vi "PSK_Error_Analysis.vi"() -> ()   [LabVIEW 2014]
uses:
  <vilib>/addons/Modulation/Digital/General/MT Generate Bits (Galois, PN Order).vi
  <vilib>/addons/Modulation/Digital/Support/Common/Validators/mod_Generate Bits Validate.vi
  <vilib>/addons/Modulation/Analog/support/mod_Set Error Source.vi
  <vilib>/addons/Modulation/Digital/General/subVIs/mod_Generate Bits PN Sequence.vi
  <vilib>/addons/Modulation/niDMT.lvlib
panel:
  in  "Packet Parameters in":T1={"Length of sync sequence (50)"=50, "Number of message bits"=128, "Number of guardbits"=40, "Sync PN sequence order (31)"=31, "Number of header bits"=16, "Packet Pad [samples]"=0}
  out "Sync Errors":i32
  out "Bit Error Rate":dbl
  out "Payload bits transfered":i32
  in  "Test Setup":T2={"Iterations"=100, "Tx IQ Sampling\nRate [s/sec]"=400000.0} {"Tx IQ Sampling\nRate [s/sec]" format="%#.6p"}
  in  "Impairments":T3={"Delay (samples)"=9, "Eb/N0 (10 dB)"=10.0} {"Eb/N0 (10 dB)" format="%.2f"}
  out "Bit errors":i64
  out "Waveform Graph":cluster{"t0":dbl, "dt":dbl, "Y":dbl[]}[](graph)
  out "Packet Length (bits)":i32
  out "Max Xcorr Index Delayed":i32
  in  "PN sequence order (9)":i32=9 caption="Message PN sequence order"
  out "Frame Offset (measured)":i32
  out "output bit stream 2":i8[](array[numeric]) caption="Transmitted Packet"
  out "output bit stream":i8[](array[numeric]) caption="Received Packet"
  in  "filter parameters":T4={"Alpha"=0.5, "Filter Length"=6, "TX Filter"=enum."Root Raised Cos"} {"Alpha" format="%.2f"}
  in  "QPSK System Parameters":T5={"Samples per Symbol"=8, "symbol map"=[], "Differential PSK"=enum."disable", "PSK type"=0, "M-PSK"=4} {"PSK type" items=["normal", "shifted", "offset"]; "symbol map" format="%.3f"}
  out "Packet Length (samples)":i32
  out "Max Xcorr Index Ideal":i32
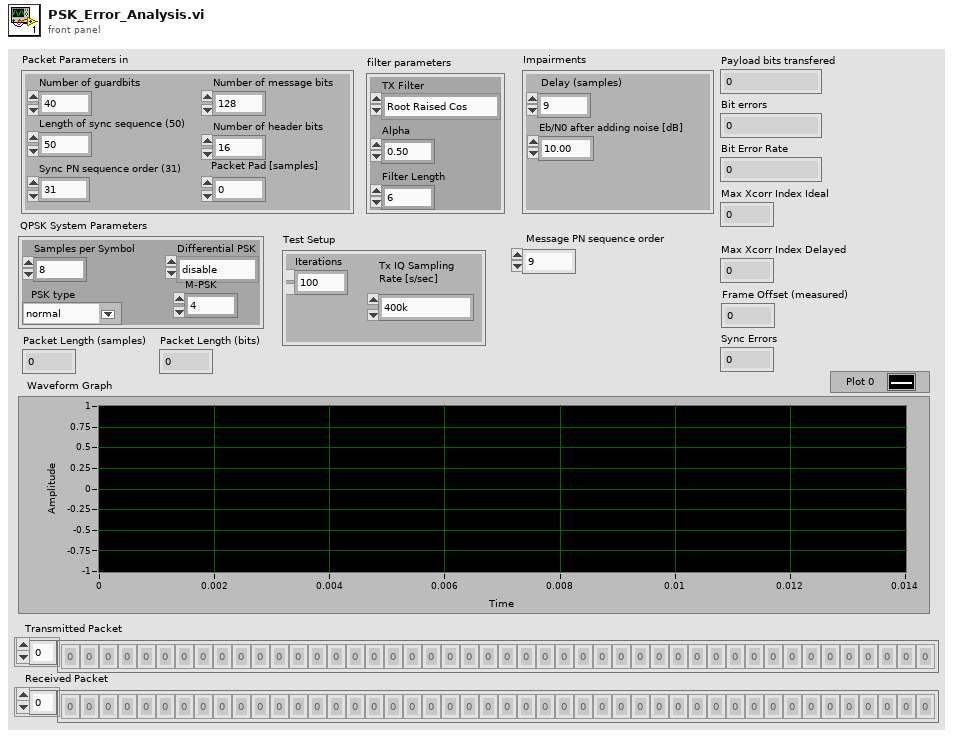
[diagram p1: front panel]
types:
  T1 = cluster{"Length of sync sequence (50)":i32, "Number of message bits":i32, "Number of guardbits":i32, "Sync PN sequence order (31)":i32, "Number of header bits":i32, "Packet Pad [samples]":i32}
  T2 = cluster{"Iterations":i32, "Tx IQ Sampling\nRate [s/sec]":dbl}
  T3 = cluster{"Delay (samples)":i32, "Eb/N0 (10 dB)":dbl}
  T4 = cluster{"Alpha":dbl, "Filter Length":i32, "TX Filter":enum16{"none", "Raised Cosine", "Root Raised Cos", "Gaussian"}}
  T5 = cluster{"Samples per Symbol":i32, "symbol map":cdb[], "Differential PSK":enum16{"disable", "enable"}, "PSK type":u16, "M-PSK":i32}
  T6 = cluster{"samples per symbol (16)":i32, "symbol map":cdb[], "differential PSK":enum16{"disable", "enable"}, "PSK type":u16}
  T7 = typedef "niAMT.lvlib/Complex Data Waveform.ctl" = cluster{"t0":dbl, "dt":dbl, "Y":cdb[]}
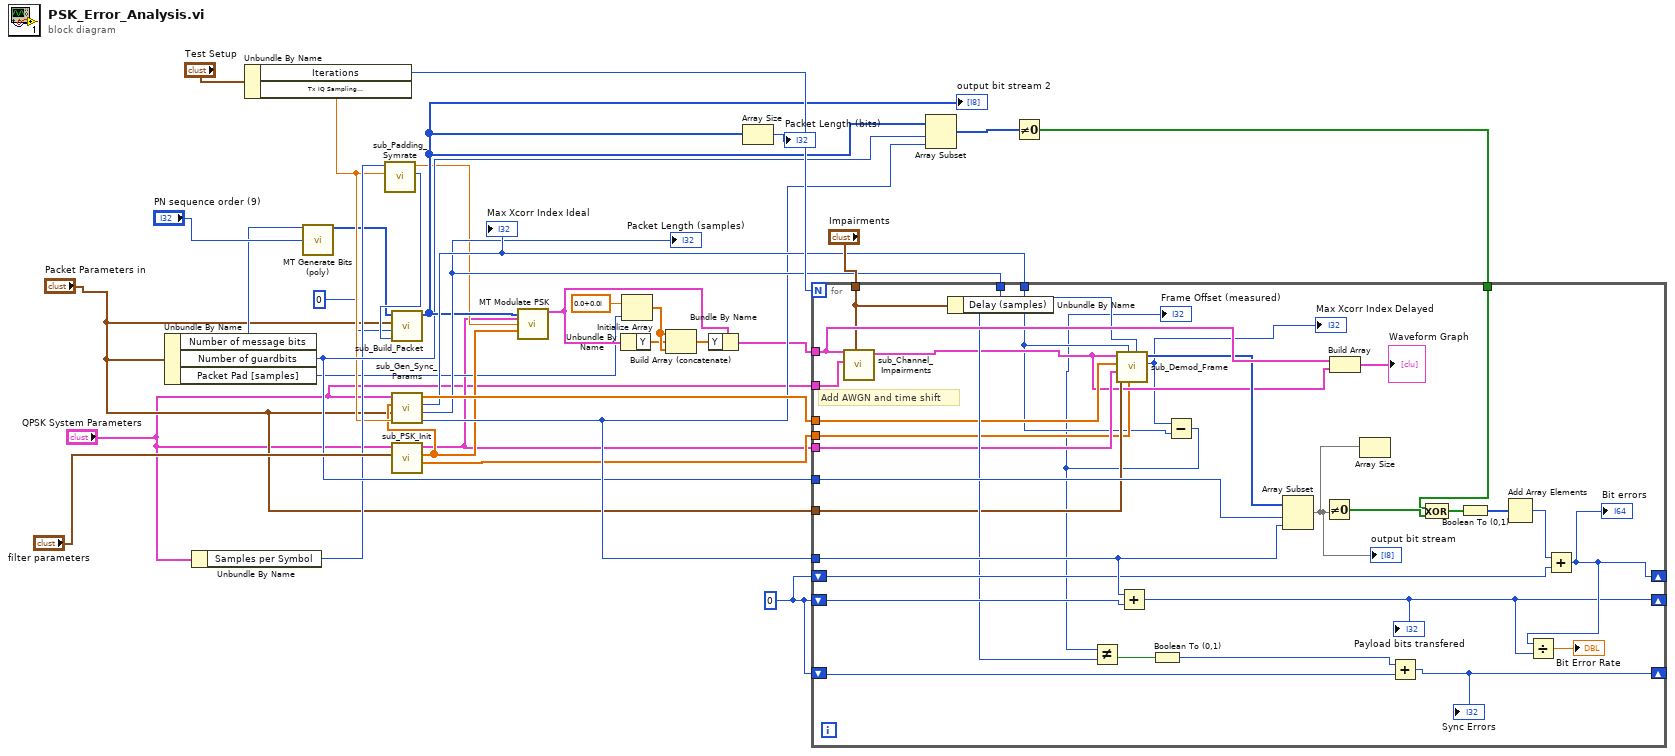
[diagram p0: block diagram]
diagram:
  w28 = i64 0 ("y")
  n1 = Unbundle By Name("Packet Parameters in") -> ("Number of message bits"=w21:i32, "Number of guardbits"=w19:i32, "Packet Pad [samples]"=w4:i32)
  n2 = Unbundle By Name("QPSK System Parameters") -> ("Samples per Symbol"=w16:i32)
  n3 = Unbundle By Name("Test Setup") -> ("Iterations"=w30:i32, "Tx IQ Sampling\nRate [s/sec]"=w14:dbl)
  n4 = call-poly <vilib>:"MT Generate Bits (poly).vi"("total bits (128)"=w21, "PN sequence order (9)"="PN sequence order (9)") -> ("output bit stream"=w13:i8[])  [unwired: 11 in, 2 out]
  n5 = call "sub_Padding_Symrate.vi"("Tx IQ Sampling\nRate [s/sec]"=w14, "Samples per Symbol"=w16) -> ("Padding Bits"=w18:i32, "Symbol Rate"=w17:dbl)  [unwired: 8 in]
  n6 = call "sub_Build_Packet.vi"("Cyclic Padding Bits"=w18, "Packet number"=i16 0, "Packet Parameters in"="Packet Parameters in", "Input Message"=w13) -> ("Packet out"=w20:i8[])  [unwired: 7 in]
  "output bit stream 2" <- w20
  n7 = call "sub_PSK_Init.vi"("filter parameters in"="filter parameters", "QPSK System Parameters in"="QPSK System Parameters") -> ("matched filter coefficients"=w15:dbl[], "pulse shaping filter coefficients"=w11:dbl[], "PSK system parameters"=w3:T6)  [unwired: 7 in]
  n8 = call "sub_Gen_Sync_Params.vi"("Tx IQ Sampling\nRate [s/sec]"=w14, "Packet Parameters in"="Packet Parameters in", "pulse shaping filter coefficients"=w11, "QPSK System Parameters in"="QPSK System Parameters") -> ("Payload length"=w23:i32, "Packet Length (samples)"=w24:i32, "Expected Xcorr Index"=w25:i32, "Sync Sequence Waveform"=w26:cdb[])  [unwired: 4 in]
  "Max Xcorr Index Ideal" <- w25
  "Packet Length (samples)" <- w24
  n9 = call <vilib>:"MT Modulate PSK.vi"("input bit stream"=w20, "PSK system parameters"=w3, "symbol rate (Hz)"=w17, "pulse shaping filter coefficients"=w11) -> ("output complex waveform"=w6:T7)  [unwired: 9 in, 2 out]
  n10 = Unbundle By Name(w6) -> ("Y"=w7:cdb[])
  n11 = Initialize Array(cdb 0.0+0.0i ("element"), w4) -> (w8:cdb[])
  n12 = Build Array (concatenate)(w8, w7, w8) -> (w10:cdb[])
  n13 = Bundle By Name(cluster=w6, "Y"=w10) -> (w5:T7)
  n14 = Array Size(array=w20) -> (size(s)=→"Packet Length (bits)":i32)
  n15 = Array Subset(array=w20, index=w19, length=w23) -> (w32:i8[])
  n16 = Not Equal To 0?(x=w32) -> (x != 0?=w29:bool[])
  n17 = for {
    N: w30 -> [_]
    tunnel: w26 -> [w45]
    tunnel: w5 -> [w48]
    tunnel: w25 -> [w37]
    tunnel: w24 -> [w44]
    tunnel: w19 -> [w65]
    tunnel: w23 -> [w63]
    shift-right: [w49] -> _
    shift-left: w28 -> [w64]
    tunnel: w29 -> [w59]
    shift-right: [w50] -> _
    shift-left: w28 -> [w57]
    shift-right: [w52] -> _
    shift-left: w28 -> [w53]
    tunnel: "Impairments" -> [w47]
    tunnel: w15 -> [w39]
    tunnel: w3 -> [w42]
    tunnel: "Packet Parameters in" -> [w41]
    tunnel: "QPSK System Parameters" -> [w35]
    # "Add AWGN and time shift"
    n18 = call "sub_Channel_Impairments.vi"("Impairments in"=w47, "QPSK System Parameters"=w35, "input complex waveform"=w48) -> ("output cluster"=w40:T7)  [unwired: 7 in, 1 out]
    n19 = Unbundle By Name(w47) -> ("Delay (samples)"=w46:i32)
    n20 = call "sub_Demod_Frame.vi"("Packet Length [samples]"=w44, "matched filter coefficients"=w39, "Expected Xcorr Index"=w37, "Packet Parameters in"=w41, "PSK system parameters"=w42, "Sync Sequence Waveform"=w45, "Input Complex Waveform"=w40) -> ("Max Xcorr Index"=w38:i32, "output bit stream"=w43:i8[])  [unwired: 3 in]
    "Max Xcorr Index Delayed" <- w38
    n21 = Add(x=w63, y=w64) -> (x+y=w49:i64)
    "Payload bits transfered" <- w49
    n22 = Subtract(x=w38, y=w37) -> (x-y=w36:i32)
    "Frame Offset (measured)" <- w36
    n23 = Not Equal?(x=w36, y=w46) -> (x != y?=w55:bool)
    n24 = Boolean To (0,1)(Boolean=w55) -> (0, 1=w54:i16)
    n25 = Array Subset(array=w43, index=w65, length=w63) -> (w56:i8[])
    "output bit stream" <- w56
    n26 = Not Equal To 0?(x=w56) -> (x != 0?=w60:bool[])
    n27 = Build Array(w48, w40) -> (→"Waveform Graph":T7[])
    n28 = Array Size(array=w56) -> ()  [unwired: 1 out]
    n29 = Add(x=w54, y=w53) -> (x+y=w52:i64)
    "Sync Errors" <- w52
    n30 = Exclusive Or(1:w60, 2:w59) -> (0:w61:bool[])
    n31 = Boolean To (0,1)(Boolean=w61) -> (0, 1=w62:i16[])
    n32 = Add Array Elements(numeric array=w62) -> (sum=w58:i16)
    n33 = Add(x=w58, y=w57) -> (x+y=w50:i64)
    "Bit errors" <- w50
    n34 = Divide(x=w50, y=w49) -> (x/y=→"Bit Error Rate":dbl)
  }
